vi "Configure Control Mode.vi"(0 "VISA resource name":refnum<visa-resource-name>, 1 "Enable Power-up (F: Disable)":bool, 2 "Setpoint Change Delay (25sec)":i32=25 min=1 max=255 step=1, 3 "Output (0: sample heater)":u16(ring) items=["sample heater", "output 1 (warm-up heater) ", "output 2 (analog/still)"], 5 "Channel (1:1)":u16(ring)=1 items=["1"=1, "2"=2, "3"=3, "4"=4, "5"=5, "6"=6, "7"=7, "8"=8, "9"=9, "10"=10, "11"=11, "12"=12, "13"=13, "14"=14, "15"=15, "16"=16, "A (Control Input)"=17], 7 "Output Mode (0: Off)":u16(ring) items=["Off", "Monitor Out", "Open Loop (Manual)", "Zone", "Still", "Closed Loop (PID)", "Warm-up"], 9 "Polarity (0: Unipolar)":u16(ring) items=["Unipolar", "Bipolar"], 11 "error in (no error)":errorcluster, 12 "Filtered Readings (0: Unfiltered)":u16(ring) items=["Unfiltered", "Filtered"], 13 "Warmup Control (0: Auto off)":u16(ring) items=["Auto off", "Continuous"], 14 "Warmup % (50%)":dbl=50.0 min=0.0 max=100.0 step=1.0) -> (4 "VISA resource name out":refnum<visa-resource-name>, 15 "error out":errorcluster)   [LabVIEW 2019, in "Lake Shore 372.lvlib"]
doc: "Configures the output mode for control for the sample heater, warm-up heater, and analog/still. The VI combines <B>OUTMODE</B> and <B>WARMUP</B> to properly configure the the output to control. Please refer to Model 372 manual for further explanations."
uses:
  Lake Shore 372.lvlib
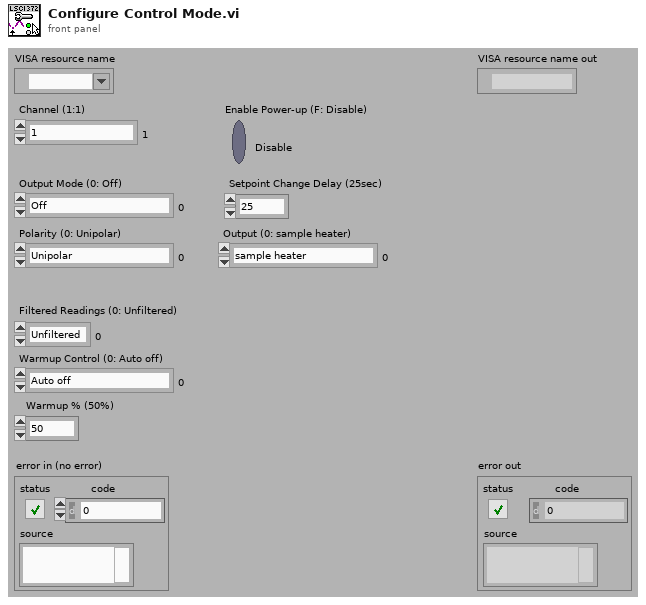
[diagram p1: front panel]
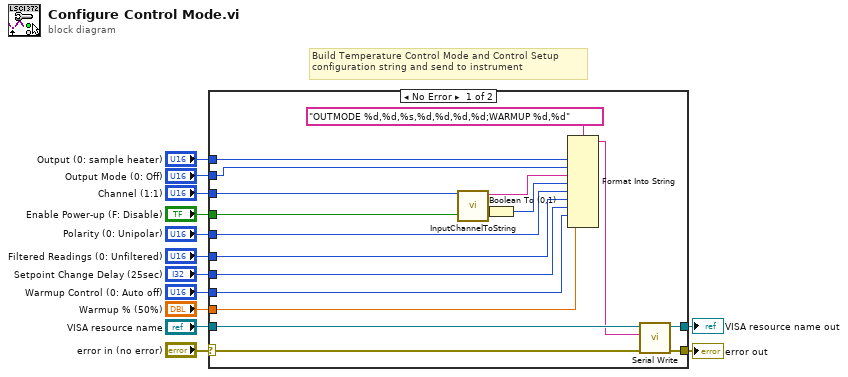
[diagram p0: block diagram]
diagram:
  # "Build Temperature Control Mode and Control Setup\nconfiguration string and send to instrument"
  n1 = case shown="No Error" "error in (no error)" {
    selector: "error in (no error)" -> [w20 w32]
    tunnel: "VISA resource name" -> [w30 w31]
    tunnel: [w29 w32] -> w12
    tunnel: [w28 w31] -> w11
    tunnel: "Warmup Control (0: Auto off)" -> [w23 _]
    tunnel: "Warmup % (50%)" -> [w22 _]
    tunnel: "Output (0: sample heater)" -> [w21 _]
    tunnel: "Output Mode (0: Off)" -> [w19 _]
    tunnel: "Channel (1:1)" -> [w18 _]
    tunnel: "Enable Power-up (F: Disable)" -> [w17 _]
    tunnel: "Polarity (0: Unipolar)" -> [w16 _]
    tunnel: "Filtered Readings (0: Unfiltered)" -> [w15 _]
    tunnel: "Setpoint Change Delay (25sec)" -> [w14 _]
    frame No Error {
      n2 = call "InputChannelToString.vi"("Channel (1)"=w18) -> ("Channel Str"=w25:string)  [unwired: 10 in]
      n3 = Boolean To (0,1)(Boolean=w17) -> (0, 1=w24:i16)
      n4 = Format Into String(format string="OUTMODE %d,%d,%s,%d,%d,%d,%d;WARMUP %d,%d", w21, w19, w25, w24, w16, w15, w14, w23, w22) -> (resulting string=w26:string)  [unwired: 2 in, 1 out]
      n5 = call "Serial Write.vi"("error in (no error)"=w20, "Write Buffer (\"\")"=w26, "VISA resource name"=w30) -> ("error out"=w29:errorcluster, "VISA resource name out"=w28:refnum<visa-resource-name>)  [unwired: 6 in, 1 out]
    }
    frame Error {
    }
  }
  "error out" <- w12
  "VISA resource name out" <- w11
